vi "Read NI 9213.vi"(8 "error in":errorcluster, 11 "NI 9213 in":refnum<class "NI 9213.lvclass">) -> (0 "error out":errorcluster, 1 "module settings":T4={"conversion time"=enum."High Resolution", "open thermocouple detection"=FALSE}, 2 "channel settings":T1[](array[typedef]), 3 "NI 9213 out":refnum<class "NI 9213.lvclass">)   [LabVIEW 2020, in "Scan Engine Scripting.lvlib" / "NI 9213.lvclass"]
doc: "Returns the channel settings of a NI-9213 analog input module that can be edited and then used to create a new module instance to set into a slot."
uses:
  NI 9213.lvclass
  NI 9213 Settings.ctl
  NI 9213 Conversion Time.ctl
  Mode Classes/Controls/thermocouple channel settings.ctl
  Channel Classes/Thermocouple Channel/Thermocouple Type.ctl
  Channel Classes/Thermocouple Channel/Measurement Units.ctl
  Channel Classes/Thermocouple Channel/Thermocouple Channel.lvclass
  Scan Engine Scripting.lvlib
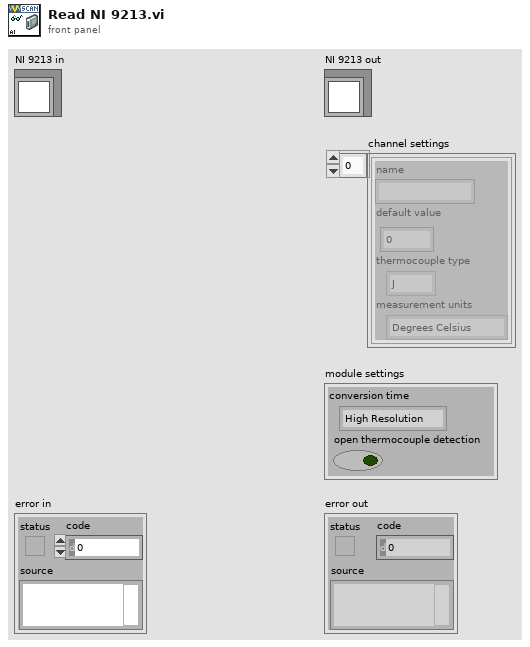
[diagram p1: front panel]
types:
  T1 = typedef "Scan Engine Scripting.lvlib/thermocouple channel settings.ctl" = cluster{"name":string, "default value":dbl, "thermocouple type":T2, "measurement units":T3}
  T2 = typedef "Scan Engine Scripting.lvlib/Thermocouple Channel.lvclass/Thermocouple Type.ctl" = enum16{"J", "K", "T", "E", "R", "S", "N", "B"}
  T3 = typedef "Scan Engine Scripting.lvlib/Thermocouple Channel.lvclass/Measurement Units.ctl" = enum16{"Raw Volts", "Degrees Kelvin", "Degrees Celsius", "Degrees Fahrenheit", "Degrees Rankine"}
  T4 = typedef "Scan Engine Scripting.lvlib/NI 9213.lvclass/NI 9213 Settings.ctl" = cluster{"conversion time":T5, "open thermocouple detection":bool}
  T5 = typedef "Scan Engine Scripting.lvlib/NI 9213.lvclass/NI 9213 Conversion Time.ctl" = enum16{"High Speed", "High Resolution"}
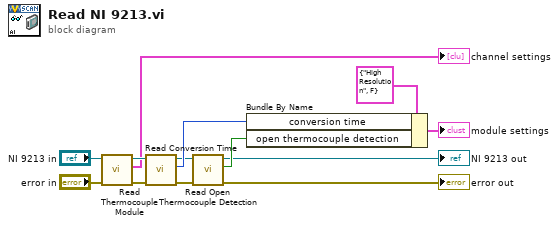
[diagram p0: block diagram]
diagram:
  n1 = call-dynamic "Read Thermocouple Module.vi"("error in"="error in", "module in"="NI 9213 in") -> ("error out"=w11:errorcluster, "channel settings"=→"channel settings":T1[], "module out"=w12:refnum<class "NI 9213.lvclass">)  [unwired: 7 in]
  n2 = call-dynamic "Read Conversion Time.vi"("error in"=w11, "NI 9213 in"=w12) -> ("error out"=w7:errorcluster, "conversion time"=w8:T5, "NI 9213 out"=w6:refnum<class "NI 9213.lvclass">)  [unwired: 7 in]
  n3 = call "Read Open Thermocouple Detection.vi"("error in"=w7, "NI 9213 in"=w6) -> ("error out"=→"error out":errorcluster, "open thermocouple detection"=w5:bool, "NI 9213 out"=→"NI 9213 out":refnum<class "NI 9213.lvclass">)  [unwired: 7 in]
  n4 = Bundle By Name(cluster=T4 {"conversion time"=enum."High Resolution", "open thermocouple detection"=FALSE} ("module settings"), "conversion time"=w8, "open thermocouple detection"=w5) -> (→"module settings":T4)
